vi "Event0--Const.vi"() -> (3 "Event Command":string)   [LabVIEW 2017, in "Communications Library.lvlib"]
uses:
  Communications Library.lvlib
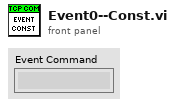
[diagram p1: front panel]
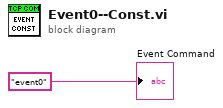
[diagram p0: block diagram]
diagram:
  "Event Command" <- "event0" ("data in")
